vi "resetHardpoints.vi"(8 "error in (no error)":errorcluster, 9 "TriggerIRQ":bool, 10 "WaitForTrigger":bool, 11 "Model in":refnum<class "Model.lvclass">) -> (0 "error out":errorcluster, 3 "Model out":refnum<class "Model.lvclass">)   [LabVIEW 2016, in "Model.lvclass"]
uses:
  Model.lvclass
  Model.lvclass/Model.ctl
  ILCCommunications/ILCCommunications.lvclass
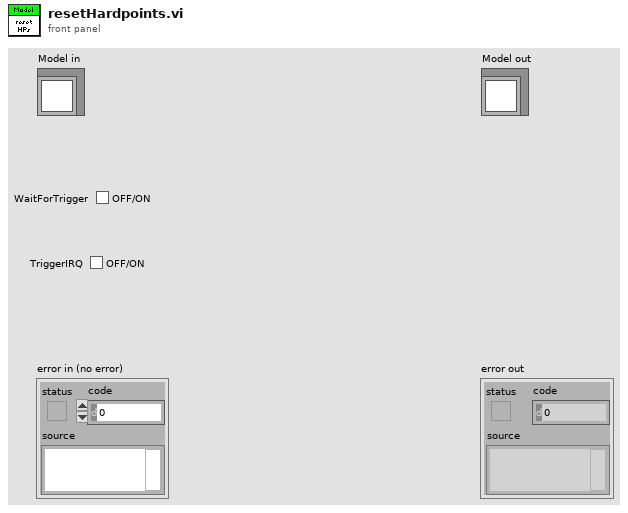
[diagram p1: front panel]
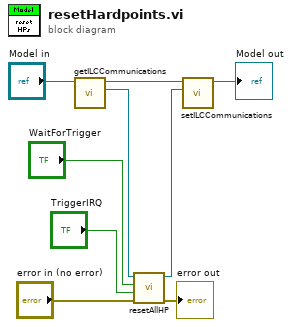
[diagram p0: block diagram]
diagram:
  n1 = call "getILCCommunications.vi"("Model in"="Model in") -> ("ILCCommunications"=w8:refnum<class "ILCCommunications.lvclass">, "Model out"=w3:refnum<class "Model.lvclass">)  [unwired: 9 in]
  n2 = call "resetAllHP.vi"("error in (no error)"="error in (no error)", "TriggerIRQ"="TriggerIRQ", "WaitForTrigger"="WaitForTrigger", "ILCCommunications in"=w8) -> ("error out"=→"error out":errorcluster, "ILCCommunications out"=w4:refnum<class "ILCCommunications.lvclass">)  [unwired: 6 in]
  n3 = call "setILCCommunications.vi"("ILCCommunications"=w4, "Model in"=w3) -> ("Model out"=→"Model out":refnum<class "Model.lvclass">)  [unwired: 9 in]
